vi "Multiply.vi"(1 "Scalar":sgl, 2 "Vector in":refnum<class "Vector2.lvclass">) -> (0 "Vector out":refnum<class "Vector2.lvclass">)   [LabVIEW 2022 SP3, in "Vector2.lvclass"]
uses:
  Vector2.lvclass
  Vector2.lvclass/Vector2.ctl
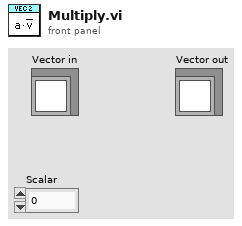
[diagram p1: front panel]
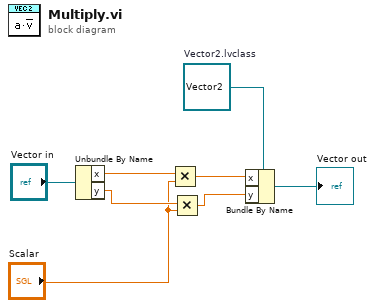
[diagram p0: block diagram]
diagram:
  w4 = refnum<class "Vector2.lvclass"> refnum  # Vector2.lvclass
  n1 = Unbundle By Name("Vector in") -> ("x"=w7:sgl, "y"=w6:sgl)
  n2 = Multiply(x=w7, y="Scalar") -> (x*y=w3:sgl)
  n3 = Multiply(x=w6, y="Scalar") -> (x*y=w2:sgl)
  n4 = Bundle By Name(cluster=w4, "x"=w3, "y"=w2) -> (→"Vector out":refnum<class "Vector2.lvclass">)
